vi "ThrowGenericError.vi"(8 "error in (no error)":errorcluster, 9 "Invoke?":bool, 10 "Error info":string, 11 "TheError":string) -> (0 "error out":errorcluster)   [LabVIEW 2017]
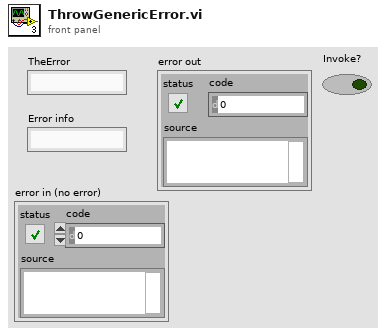
[diagram p1: front panel]
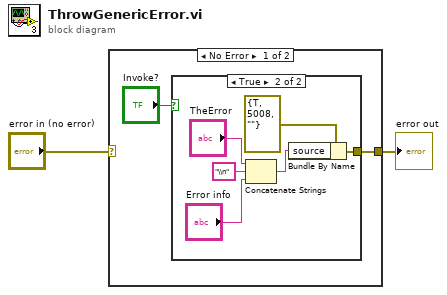
[diagram p0: block diagram]
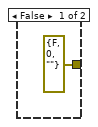
[diagram p2: hidden frame]
diagram:
  n1 = case shown="No Error" "error in (no error)" {
    selector: "error in (no error)" -> [_ w12]
    tunnel: [w4 w12] -> w2
    frame No Error {
      n2 = case shown="True" "Invoke?" {
        tunnel: [errorcluster {"status"=FALSE, "code"=0, "source"=""} ("error out") w6] -> w4
        frame False {
        }
        frame True {
          n3 = Concatenate Strings("TheError", "\\n" ("string"), "Error info") -> (w7:string)
          n4 = Bundle By Name(cluster=errorcluster {"status"=TRUE, "code"=5008, "source"=""} ("error in (no error)"), "source"=w7) -> (w6:errorcluster)
        }
      }
    }
    frame Error {
    }
  }
  "error out" <- w2
